vi "Scale sensor data.vi"(7 "Channel type":T1=enum."Flow meter", 11 "RAW Value":dbl) -> (2 "Type name":string, 3 "Scaled value":dbl)   [LabVIEW 2015]
uses:
  Channel type.ctl
  <vilib>/ptbypt/NI_PtbyPt.lvlib
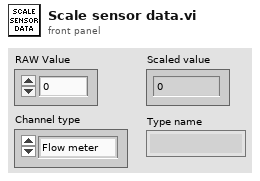
[diagram p1: front panel]
types:
  T1 = typedef "Channel type.ctl" = enum16{"Volts", "Flow meter", "Tank pressure", "Dewar level", "Raw ADC"}
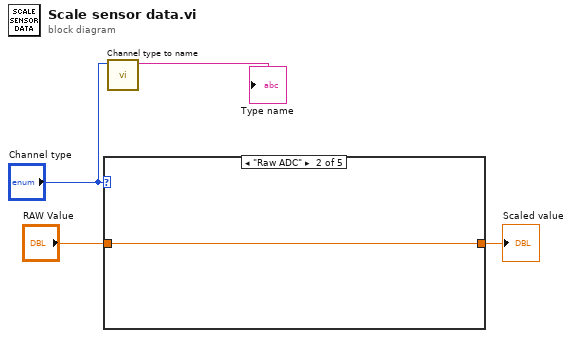
[diagram p0: block diagram]
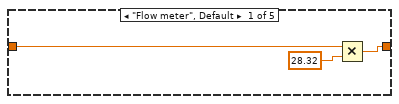
[diagram p2: hidden frame]
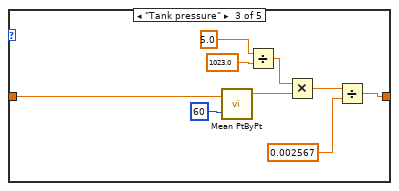
[diagram p3: hidden frame]
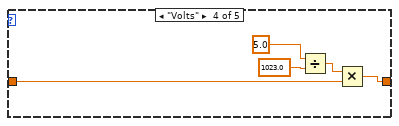
[diagram p4: hidden frame]
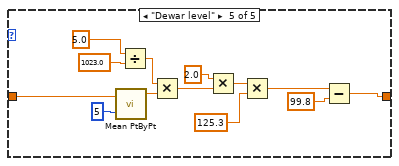
[diagram p5: hidden frame]
diagram:
  n1 = case shown="\"Raw ADC\"" "Channel type" {
    tunnel: [w5 w8 w9 w18 w23] -> w4
    tunnel: "RAW Value" -> [w6 w8 w15 w19 w34]
    frame "Flow meter", Default {
      n2 = Multiply(x=w6, y=28.32) -> (x*y=w5:dbl)
    }
    frame "Raw ADC" {
    }
    frame "Tank pressure" {
      n3 = call <vilib>:"Mean PtByPt.vi"("x"=w15, "sample length"=60) -> ("mean"=w16:dbl)  [unwired: 2 in, 1 out]
      n4 = Divide(x=5.0, y=1023.0) -> (x/y=w12:dbl)
      n5 = Multiply(x=w12, y=w16) -> (x*y=w10:dbl)
      n6 = Divide(x=w10, y=0.002567) -> (x/y=w9:dbl)
    }
    frame "Volts" {
      n7 = Divide(x=5.0, y=1023.0) -> (x/y=w20:dbl)
      n8 = Multiply(x=w20, y=w19) -> (x*y=w18:dbl)
    }
    frame "Dewar level" {
      n9 = call <vilib>:"Mean PtByPt.vi"("x"=w34, "sample length"=5) -> ("mean"=w31:dbl)  [unwired: 2 in, 1 out]
      n10 = Divide(x=5.0, y=1023.0) -> (x/y=w30:dbl)
      n11 = Multiply(x=w30, y=w31) -> (x*y=w24:dbl)
      n12 = Multiply(x=2.0, y=w24) -> (x*y=w26:dbl)
      n13 = Multiply(x=w26, y=125.3) -> (x*y=w28:dbl)
      n14 = Subtract(x=w28, y=99.8) -> (x-y=w23:dbl)
    }
  }
  "Scaled value" <- w4
  n15 = call "Channel type to name.vi"("Channel type"="Channel type") -> ("Name"=→"Type name":string)  [unwired: 9 in, 1 out]
